vi "Timeslot.vi"(0 "Write Req Grant Time (clocks)":u16=1000, 5 "Read Req Grant Time (clocks)":u16=5) -> (6 "Mux Select":bool=TRUE)   [LabVIEW 2013]
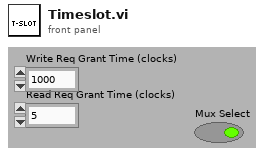
[diagram p1: front panel]
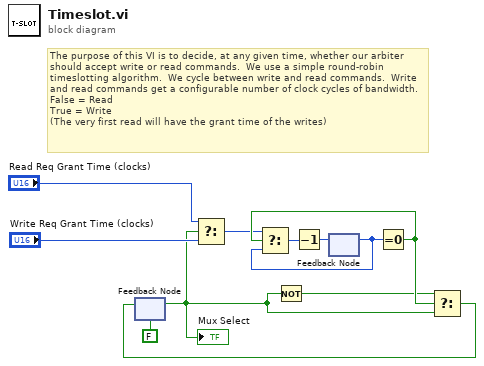
[diagram p0: block diagram]
diagram:
  # "The purpose of this VI is to decide, at any given time, whether our arbiter should accept write or read commands.  We use a simple round-robin timeslotting algorithm.  We cycle between write and read commands.  Write and read commands get a configurable number of clock cycles of bandwidth.\nFalse = Read\nTrue = Write\n(The very first read will have the grant time of the writes)"
  n1 = feedback #1 ("Cmd\nTimeslot")(FALSE ("read")) -> (w1:bool)
  "Mux Select" <- w1
  n2 = Select(t="Read Req Grant Time (clocks)", s=w1, f="Write Req Grant Time (clocks)") -> (s? t:f=w5:u16)
  n3 = Not(x=w1) -> (.not. x?=w4:bool)
  n4 = feedback #2() -> (w9:u16)  [unwired: 1 in]
  n5 = Equal To 0?(x=w9) -> (x = 0?=w6:bool)
  n6 = Select(t=w5, s=w6, f=w9) -> (s? t:f=w8:u16)
  n7 = Decrement(x=w8) -> (x-1=w7:u16)
  n8 = feedback-in #2(w7) -> ()
  n9 = Select(t=w4, s=w6, f=w1) -> (s? t:f=w10:bool)
  n10 = feedback-in #1(w10) -> ()
